vi "Export Configuration.vi"(8 "error in (no error)":errorcluster, 11 "Node Ptr":u64 format="%.0x") -> (0 "error out":errorcluster)   [LabVIEW 2024, in "Embedded TDMS Logger System Explorer.lvlib"]
doc: "Exports the current configuration of the Custom Device in the System Definition to XML - is useful for backing up specifically the configuration, for documenting it into Github, for processing/modifying it in a script."
uses:
  Embedded TDMS Logger System Explorer.lvlib
panel:
  in  "Tag":string
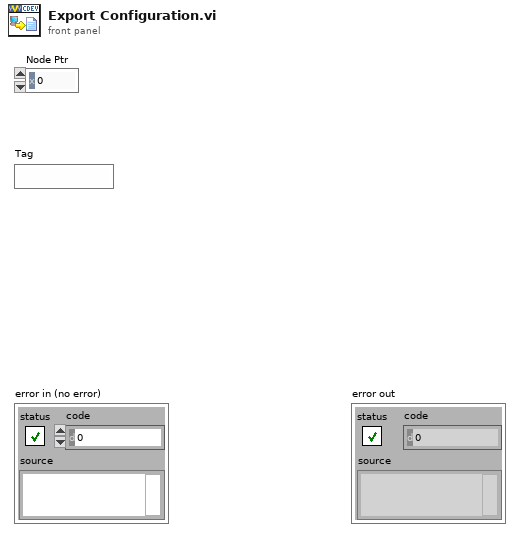
[diagram p1: front panel]
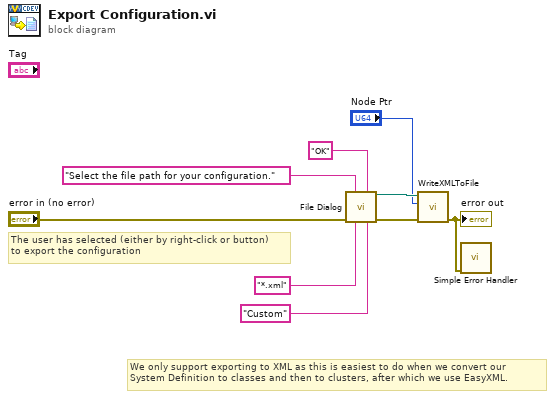
[diagram p0: block diagram]
diagram:
  # "We only support exporting to XML as this is easiest to do when we convert our \nSystem Definition to classes and then to clusters, after which we use EasyXML."
  # "The user has selected (either by right-click or button)\nto export the configuration"
  n1 = call "File Dialog"("prompt"="Select the file path for your configuration.", "button label"="OK", "error in"="error in (no error)", "pattern (all files)"="*.xml", "pattern label"="Custom") -> ("selected path"=w3:path, "error out"=w4:errorcluster)  [unwired: 7 in, 2 out]
  n2 = call "WriteXMLToFile.vi"("error in (no error)"=w4, "Node Ptr"="Node Ptr", "selected path"=w3) -> ("error out"=w2:errorcluster)  [unwired: 8 in]
  "error out" <- w2
  n3 = call <vilib>:"Simple Error Handler.vi"("error in (no error)"=w2) -> ()  [unwired: 4 in, 5 out]
